vi "stringtoin18.vi"(11 "input_string":string) -> (0 "channel":u8 format="%x", 1 "counter":u8, 2 "outputComplemented_int":i32, 3 "output_int":u32 format="%x")   [LabVIEW 2014]
panel:
  out "(hi.lo) 2":u32 format="%x"
  out "(hi.lo)":u16 format="%x"
  out "number 4":u8 format="%x"
  out "number 3":u8 format="%x"
  out "number 2":u8 format="%x"
  out "number":u8 format="%x"
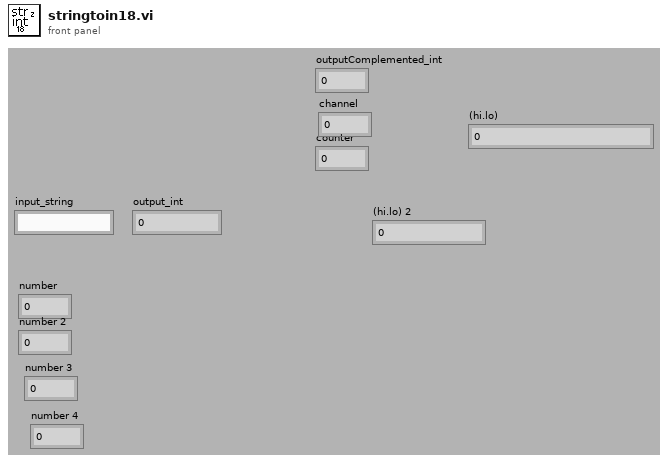
[diagram p1: front panel]
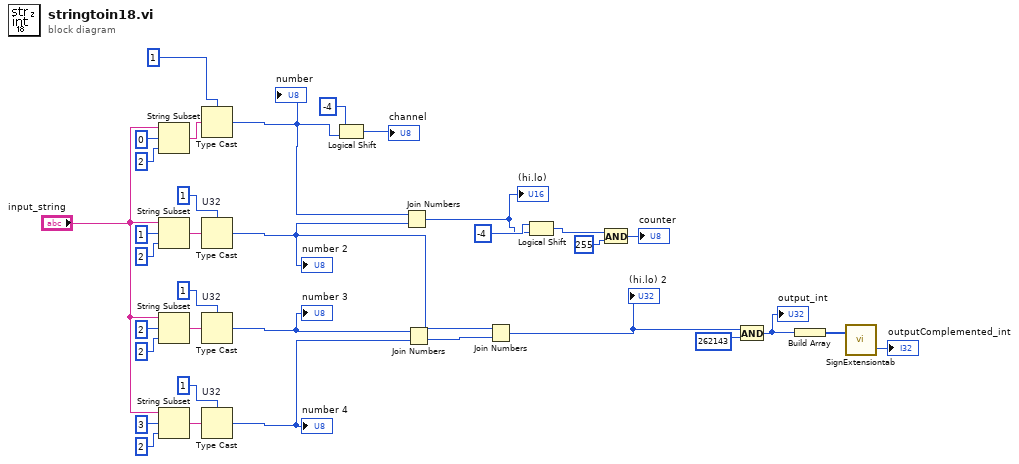
[diagram p0: block diagram]
diagram:
  n1 = String Subset(string="input_string", offset (0)=0, length (rest)=2 ("length (rest)")) -> (substring=w26:string)
  n2 = String Subset(string="input_string", offset (0)=1, length (rest)=2 ("length (rest)")) -> (substring=w25:string)
  n3 = String Subset(string="input_string", offset (0)=2, length (rest)=2 ("length (rest)")) -> (substring=w18:string)
  n4 = String Subset(string="input_string", offset (0)=3, length (rest)=2 ("length (rest)")) -> (substring=w16:string)
  n5 = Type Cast(type=u8 1 ("Numeric"), x=w26) -> (*(type *) &x=w6:u8)
  "number" <- w6
  n6 = Type Cast "U32"(type=u8 1 ("Numeric"), x=w25) -> (*(type *) &x=w29:u8)
  "number 2" <- w29
  n7 = Type Cast "U32"(type=u8 1 ("Numeric"), x=w18) -> (*(type *) &x=w32:u8)
  "number 3" <- w32
  n8 = Type Cast "U32"(type=u8 1 ("Numeric"), x=w16) -> (*(type *) &x=w31:u8)
  "number 4" <- w31
  n9 = Logical Shift(y=i16 -4, x=w6) -> (x << y=→"channel":u8)
  n10 = Join Numbers(hi=w6, lo=w29) -> ((hi.lo)=w2:u16)
  "(hi.lo)" <- w2
  n11 = Join Numbers(hi=w32, lo=w31) -> ((hi.lo)=w30:u16)
  n12 = Join Numbers(hi=w29, lo=w30) -> ((hi.lo)=w34:u32)
  "(hi.lo) 2" <- w34
  n13 = Logical Shift(y=i8 -4, x=w2) -> (x << y=w1:u16)
  n14 = And(x=w1, y=u32 255) -> (x .and. y?=→"counter":u32)
  n15 = And(x=w34, y=u32 262143) -> (x .and. y?=w9:u32)
  "output_int" <- w9
  n16 = Build Array(w9) -> (w10:u32[])
  n17 = call "SignExtensiontab.vi"("inputs"=w10) -> ("scalarOutput"=→"outputComplemented_int":i32)  [unwired: 1 in, 1 out]
